vi "Set Login Hint.vi"(10 "Login Hint":string, 11 "Request in":refnum<class "Request.lvclass">) -> (3 "Request out":refnum<class "Request.lvclass">)   [LabVIEW 2020, in "OAuth2.lvlib" / "Request.lvclass"]
doc: "Used to specify the suggested account for the user to authorize with, if already known. This can usually be left blank and is only useful when an application already knows the user's account either by previous authentication that has been saved or already specified for the user to be able to use the application."
uses:
  Request.lvclass
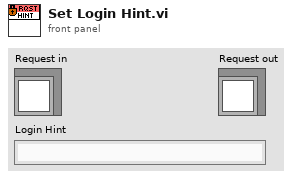
[diagram p1: front panel]
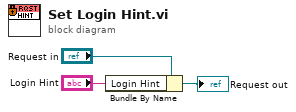
[diagram p0: block diagram]
diagram:
  n1 = Bundle By Name(cluster="Request in", "Login Hint"="Login Hint") -> (→"Request out":refnum<class "Request.lvclass">)
